vi "Read Sample Transfer.Source Sample.vi"(11 "cRIO-CO2 in":refnum<class "cRIO-CO2.lvclass">) -> (2 "Sample.lvclass":refnum<class "Sample.lvclass">, 3 "cRIO-CO2 out":refnum<class "cRIO-CO2.lvclass">)   [LabVIEW 2015, in "cRIO-Carbondioxide.lvlib" / "cRIO-CO2.lvlib" / "cRIO-CO2.lvclass"]
uses:
  cRIO-CO2.lvclass
  subs/Sample/Sample.lvclass
  cRIO-CO2.lvclass/cRIO-CO2.ctl
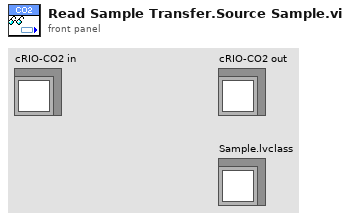
[diagram p1: front panel]
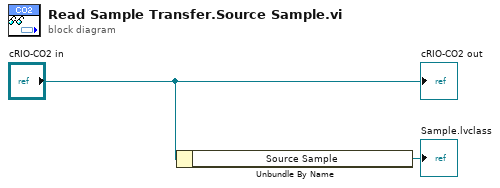
[diagram p0: block diagram]
diagram:
  n1 = Unbundle By Name("cRIO-CO2 in") -> ("Source Sample"=→"Sample.lvclass":refnum<class "Sample.lvclass">)
  "cRIO-CO2 out" <- "cRIO-CO2 in"
